vi "Encode.vi"(8 "error in (no error)":errorcluster, 10 "Data":i16[](array[numeric]), 11 "Spring Motor in":refnum<class "Spring Motor.lvclass">) -> (0 "error out":errorcluster, 2 "Message":string, 3 "Spring Motor out":refnum<class "Spring Motor.lvclass">)   [LabVIEW 2021, in "Spring Motor.lvclass"]
uses:
  Spring Motor.lvclass
  Spring Motor.lvclass/Spring Motor.ctl
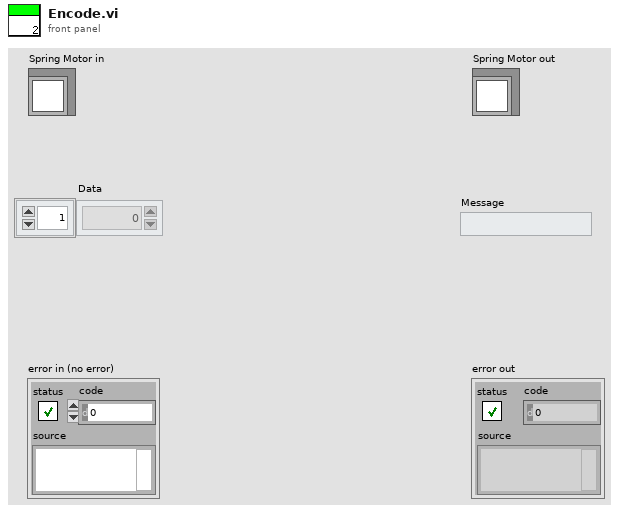
[diagram p1: front panel]
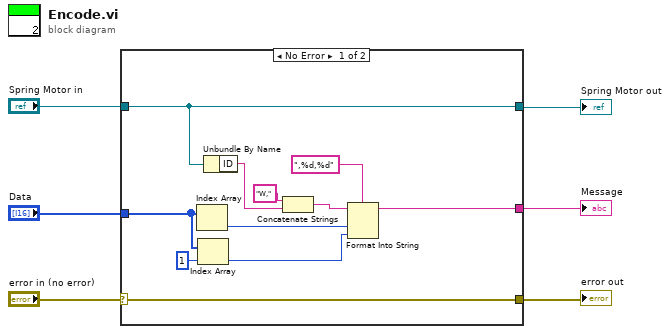
[diagram p0: block diagram]
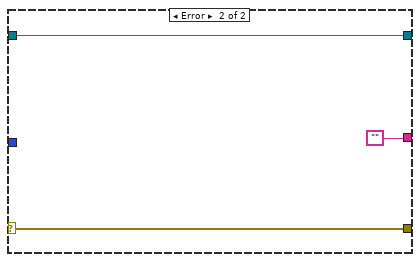
[diagram p2: hidden frame]
diagram:
  n1 = case shown="No Error" "error in (no error)" {
    selector: "error in (no error)" -> [w17 w19]
    tunnel: [w13 w20] -> w4
    tunnel: "Spring Motor in" -> [w13 w20]
    tunnel: [w17 w19] -> w3
    tunnel: "Data" -> [w9 _]
    tunnel: [w14 ""] -> w1
    frame No Error {
      n2 = Index Array(array=w9) -> (element=w16:i16)  [unwired: 1 in]
      n3 = Index Array(array=w9, index=1) -> (element=w10:i16)
      n4 = Unbundle By Name(w13) -> ("ID"=w12:string)
      n5 = Concatenate Strings("W," ("string"), w12) -> (w8:string)
      n6 = Format Into String(format string=",%d,%d", initial string=w8, w16, w10) -> (resulting string=w14:string)  [unwired: 1 in, 1 out]
    }
    frame Error {
    }
  }
  "error out" <- w3
  "Spring Motor out" <- w4
  "Message" <- w1
